vi "Reset_Instr.vi"(8 "error in (no error)":errorcluster caption="entrée d'erreur (pas d'erreur)", 11 "Class Instrument Multimeter en entrée":refnum<class "Class Instrument Multimeter.lvclass">) -> (0 "error out":errorcluster caption="sortie d'erreur", 3 "Class Instrument Multimeter en sortie":refnum<class "Class Instrument Multimeter.lvclass">)   [LabVIEW 2020, in "Library Instrument & Equipement.lvlib" / "Library Instruments.lvlib" / "Class Instrument Multimeter.lvclass"]
uses:
  Class Instrument Multimeter.lvclass
  Class Instrument Multimeter.lvclass/Class Instrument Multimeter.ctl
  Instrument (Default)/Class Instrument (Default).lvclass
  Multimeter/Multimeter (Default)/Class Multimeter (Default).lvclass
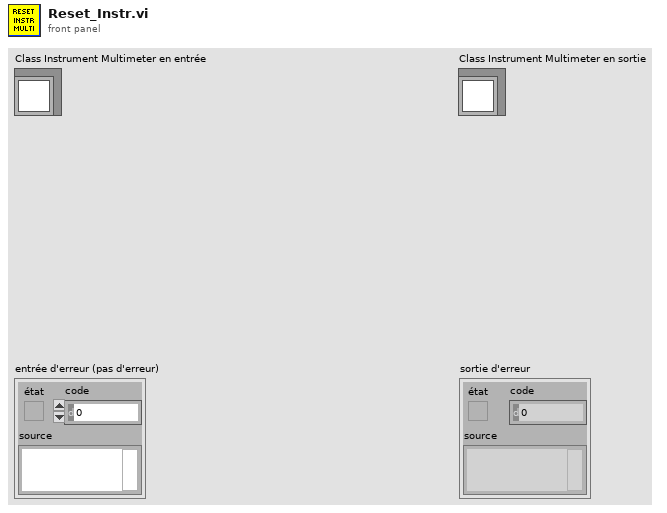
[diagram p1: front panel]
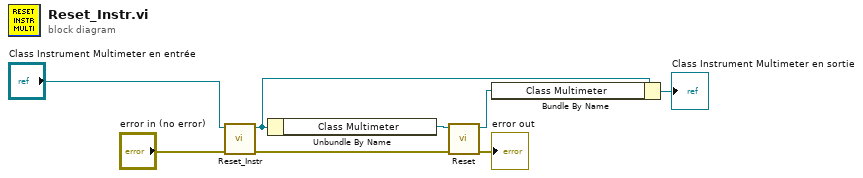
[diagram p0: block diagram]
diagram:
  n1 = call-parent "Reset_Instr.vi"("error in (no error)"="error in (no error)", "Class Instrument (Default) en entrée"="Class Instrument Multimeter en entrée") -> ("error out"=w6:errorcluster, "Class Instrument (Default) en sortie"=w3:refnum<class "Class Instrument Multimeter.lvclass">)  [unwired: 8 in]
  n2 = Unbundle By Name(w3) -> ("Class Multimeter"=w5:refnum<class "Class Multimeter (Default).lvclass">)
  n3 = call-dynamic "Reset.vi"("error in (no error)"=w6, "Class Multimeter (Default) en entrée"=w5) -> ("error out"=→"error out":errorcluster, "Class Multimeter (Default) en sortie"=w1:refnum<class "Class Multimeter (Default).lvclass">)  [unwired: 8 in]
  n4 = Bundle By Name(cluster=w3, "Class Multimeter"=w1) -> (→"Class Instrument Multimeter en sortie":refnum<class "Class Instrument Multimeter.lvclass">)
